vi "UTEXGUI.vi"(8 "ExitSendCmd":bool, 11 "UT340 Controls":T1={"High Pass On"=FALSE, "High Pass Filter (MHz)"=1, "Low Pass On"=FALSE, "Low Pass Filter (MHz)"=20, "PE Gain (dB)"=1, "Voltage"=100, "Pulse Width (ns)"=2.0, "Mode"=FALSE, "PC Gain (dB)"=1, "Trig Source"=FALSE, "Rep Rate (Hz)"=0, "PULSE"=FALSE} {"Low Pass Filter (MHz)" min=20 step=1; "High Pass Filter (MHz)" min=1 max=20 step=1; "Pulse Width (ns)" min=2.0 max=71.75; "Voltage" min=100 max=250 step=2; "PC Gain (dB)" min=0 max=63 step=1; "PE Gain (dB)" min=-6 max=57 step=1}) -> ()   [LabVIEW 2022 SP3]
uses:
  Controls/UTEX Controls.ctl
  PulserGlobals.vi
panel:
  out "error out":errorcluster
  in  "error in":errorcluster
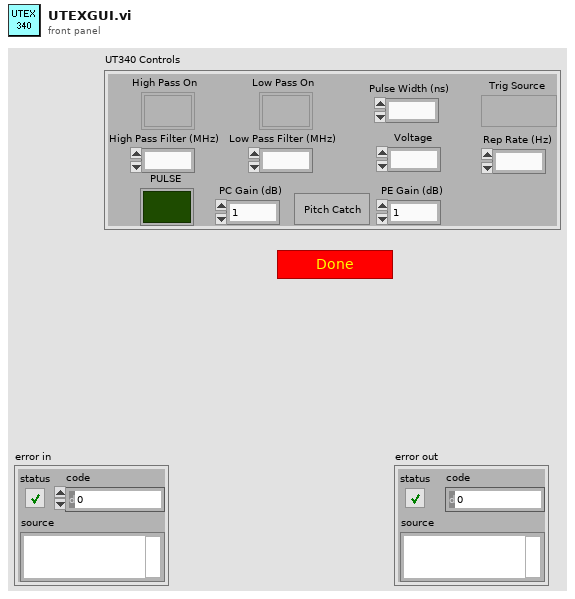
[diagram p1: front panel]
types:
  T1 = typedef "UTEX Controls.ctl" = cluster{"High Pass On":bool, "High Pass Filter (MHz)":i16, "Low Pass On":bool, "Low Pass Filter (MHz)":i16, "PE Gain (dB)":i16, "Voltage":i16, "Pulse Width (ns)":dbl, "Mode":bool, "PC Gain (dB)":i16, "Trig Source":bool, "Rep Rate (Hz)":i16, "PULSE":bool}
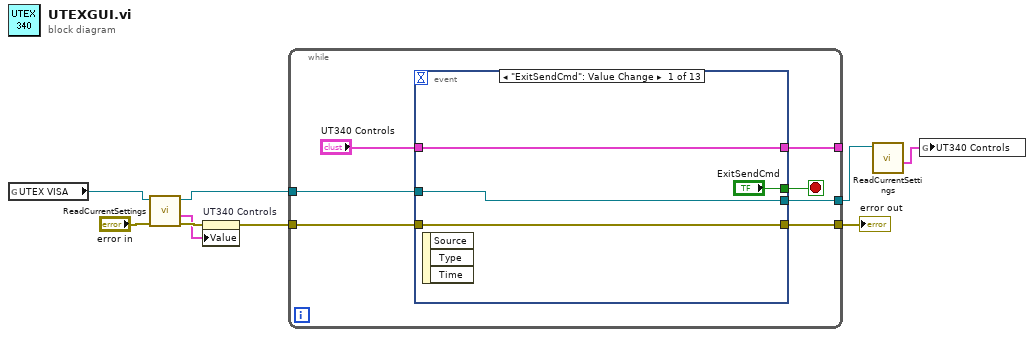
[diagram p0: block diagram]
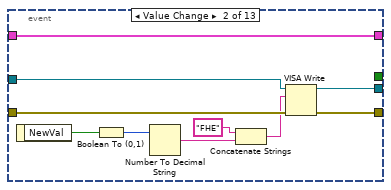
[diagram p2: hidden frame]
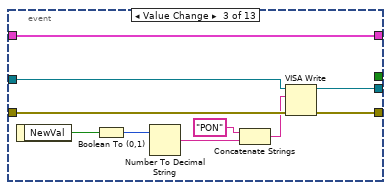
[diagram p3: hidden frame]
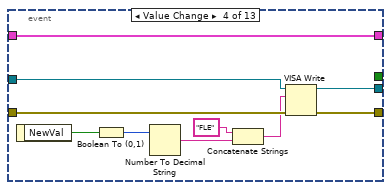
[diagram p4: hidden frame]
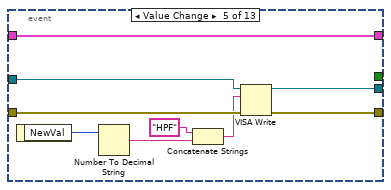
[diagram p5: hidden frame]
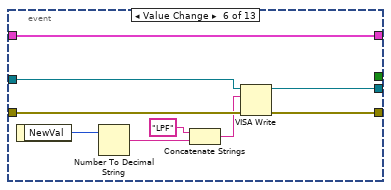
[diagram p6: hidden frame]
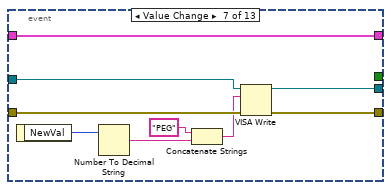
[diagram p7: hidden frame]
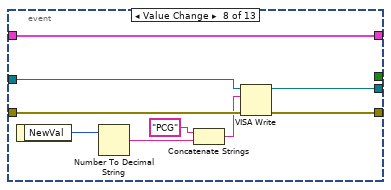
[diagram p8: hidden frame]
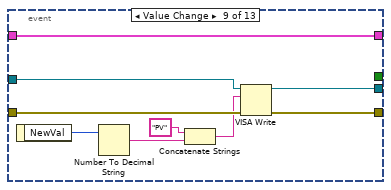
[diagram p9: hidden frame]
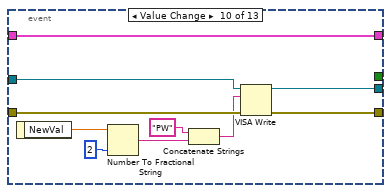
[diagram p10: hidden frame]
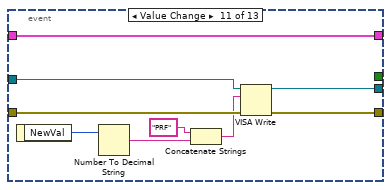
[diagram p11: hidden frame]
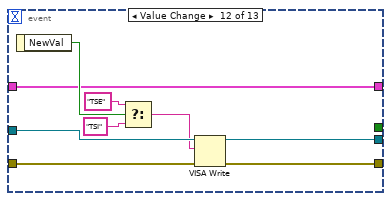
[diagram p12: hidden frame]
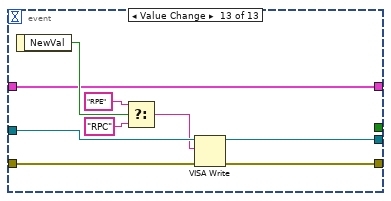
[diagram p13: hidden frame]
diagram:
  n1 = global read "PulserGlobals.vi" "UTEX VISA"() -> (w2:refnum<visa-resource-name>)
  n2 = call "ReadCurrentSettings.vi"("error in (no error)"="error in", "VISA Refnum in"=w2) -> ("error out"=w7:errorcluster, "UT340 Controls"=w4:T1, "VISA Refnum out"=w1:refnum<visa-resource-name>)  [unwired: 7 in]
  n3 = property on="UT340 Controls" class="Clust (strict)"(error in=w7, "Value"=w4) -> (error out=w8:errorcluster)  [unwired: 1 in, 1 out]
  n4 = while {
    tunnel: w8 -> [w15]
    tunnel: w1 -> [w14]
    tunnel: [w13] -> w5
    tunnel: [w12] -> w9
    tunnel: [w10] -> _
    stop <- w11 stop-if-true
    n5 = event shown="[0] \"ExitSendCmd\": Value Change" {
      selector: _ -> [_ _ _ _ _ _ _ _ _ _ _ _ _]
      dyn-events: _ -> [_ _ _ _ _ _ _ _ _ _ _ _ _]
      timeout: _ -> [_ _ _ _ _ _ _ _ _ _ _ _ _]
      tunnel: "UT340 Controls" -> [w17 w21 w31 w41 w51 w60 w69 w78 w87 w96 w106 w115 w124]
      tunnel: w15 -> [w19 w30 w40 w50 w59 w68 w77 w86 w95 w105 w114 w123 w132]
      tunnel: w14 -> [w20 w29 w39 w49 w58 w67 w76 w85 w94 w104 w113 w122 w131]
      tunnel: [w20 w28 w38 w48 w57 w66 w75 w84 w93 w103 w112 w121 w130] -> w13
      tunnel: [w19 w27 w37 w47 w56 w65 w74 w83 w92 w102 w111 w120 w129] -> w12
      tunnel: ["ExitSendCmd" _ _ _ _ _ _ _ _ _ _ _ _] -> w11
      tunnel: [w17 w21 w31 w41 w51 w60 w69 w78 w87 w96 w106 w115 w124] -> w10
      event "ExitSendCmd": Value Change {
        n6 = event-data() -> ()  [unwired: 1 in, 3 out]
      }
      event Value Change {
        n7 = event-data() -> ("NewVal"=w26:bool)  [unwired: 1 in]
        n8 = Boolean To (0,1)(Boolean=w26) -> (0, 1=w22:i16)
        n9 = Number To Decimal String(number=w22) -> (decimal integer string=w24:string)  [unwired: 1 in]
        n10 = Concatenate Strings("FHE" ("string"), w24) -> (w23:string)
        n11 = VISA Write(VISA resource name=w29, write buffer=w23, error in (no error)=w30) -> (VISA resource name out=w28:refnum<visa-resource-name>, error out=w27:errorcluster)  [unwired: 1 out]
      }
      event Value Change {
        n12 = event-data() -> ("NewVal"=w36:bool)  [unwired: 1 in]
        n13 = Boolean To (0,1)(Boolean=w36) -> (0, 1=w32:i16)
        n14 = Number To Decimal String(number=w32) -> (decimal integer string=w34:string)  [unwired: 1 in]
        n15 = Concatenate Strings("PON" ("string"), w34) -> (w33:string)
        n16 = VISA Write(VISA resource name=w39, write buffer=w33, error in (no error)=w40) -> (VISA resource name out=w38:refnum<visa-resource-name>, error out=w37:errorcluster)  [unwired: 1 out]
      }
      event Value Change {
        n17 = event-data() -> ("NewVal"=w46:bool)  [unwired: 1 in]
        n18 = Boolean To (0,1)(Boolean=w46) -> (0, 1=w42:i16)
        n19 = Number To Decimal String(number=w42) -> (decimal integer string=w44:string)  [unwired: 1 in]
        n20 = Concatenate Strings("FLE" ("string"), w44) -> (w43:string)
        n21 = VISA Write(VISA resource name=w49, write buffer=w43, error in (no error)=w50) -> (VISA resource name out=w48:refnum<visa-resource-name>, error out=w47:errorcluster)  [unwired: 1 out]
      }
      event Value Change {
        n22 = event-data() -> ("NewVal"=w55:i16)  [unwired: 1 in]
        n23 = Number To Decimal String(number=w55) -> (decimal integer string=w53:string)  [unwired: 1 in]
        n24 = Concatenate Strings("HPF" ("string"), w53) -> (w52:string)
        n25 = VISA Write(VISA resource name=w58, write buffer=w52, error in (no error)=w59) -> (VISA resource name out=w57:refnum<visa-resource-name>, error out=w56:errorcluster)  [unwired: 1 out]
      }
      event Value Change {
        n26 = event-data() -> ("NewVal"=w64:i16)  [unwired: 1 in]
        n27 = Number To Decimal String(number=w64) -> (decimal integer string=w62:string)  [unwired: 1 in]
        n28 = Concatenate Strings("LPF" ("string"), w62) -> (w61:string)
        n29 = VISA Write(VISA resource name=w67, write buffer=w61, error in (no error)=w68) -> (VISA resource name out=w66:refnum<visa-resource-name>, error out=w65:errorcluster)  [unwired: 1 out]
      }
      event Value Change {
        n30 = event-data() -> ("NewVal"=w73:i16)  [unwired: 1 in]
        n31 = Number To Decimal String(number=w73) -> (decimal integer string=w71:string)  [unwired: 1 in]
        n32 = Concatenate Strings("PEG" ("string"), w71) -> (w70:string)
        n33 = VISA Write(VISA resource name=w76, write buffer=w70, error in (no error)=w77) -> (VISA resource name out=w75:refnum<visa-resource-name>, error out=w74:errorcluster)  [unwired: 1 out]
      }
      event Value Change {
        n34 = event-data() -> ("NewVal"=w82:i16)  [unwired: 1 in]
        n35 = Number To Decimal String(number=w82) -> (decimal integer string=w80:string)  [unwired: 1 in]
        n36 = Concatenate Strings("PCG" ("string"), w80) -> (w79:string)
        n37 = VISA Write(VISA resource name=w85, write buffer=w79, error in (no error)=w86) -> (VISA resource name out=w84:refnum<visa-resource-name>, error out=w83:errorcluster)  [unwired: 1 out]
      }
      event Value Change {
        n38 = event-data() -> ("NewVal"=w91:i16)  [unwired: 1 in]
        n39 = Number To Decimal String(number=w91) -> (decimal integer string=w89:string)  [unwired: 1 in]
        n40 = Concatenate Strings("PV" ("string"), w89) -> (w88:string)
        n41 = VISA Write(VISA resource name=w94, write buffer=w88, error in (no error)=w95) -> (VISA resource name out=w93:refnum<visa-resource-name>, error out=w92:errorcluster)  [unwired: 1 out]
      }
      event Value Change {
        n42 = event-data() -> ("NewVal"=w101:dbl)  [unwired: 1 in]
        n43 = Number To Fractional String(number=w101, precision (6)=i16 2) -> (F-format string=w99:string)  [unwired: 2 in]
        n44 = Concatenate Strings("PW" ("string"), w99) -> (w98:string)
        n45 = VISA Write(VISA resource name=w104, write buffer=w98, error in (no error)=w105) -> (VISA resource name out=w103:refnum<visa-resource-name>, error out=w102:errorcluster)  [unwired: 1 out]
      }
      event Value Change {
        n46 = event-data() -> ("NewVal"=w110:i16)  [unwired: 1 in]
        n47 = Number To Decimal String(number=w110) -> (decimal integer string=w108:string)  [unwired: 1 in]
        n48 = Concatenate Strings("PRF" ("string"), w108) -> (w107:string)
        n49 = VISA Write(VISA resource name=w113, write buffer=w107, error in (no error)=w114) -> (VISA resource name out=w112:refnum<visa-resource-name>, error out=w111:errorcluster)  [unwired: 1 out]
      }
      event Value Change {
        n50 = event-data() -> ("NewVal"=w119:bool)  [unwired: 1 in]
        n51 = Select(t="TSE" ("string"), s=w119, f="TSI") -> (s? t:f=w118:string)
        n52 = VISA Write(VISA resource name=w122, write buffer=w118, error in (no error)=w123) -> (VISA resource name out=w121:refnum<visa-resource-name>, error out=w120:errorcluster)  [unwired: 1 out]
      }
      event Value Change {
        n53 = event-data() -> ("NewVal"=w128:bool)  [unwired: 1 in]
        n54 = Select(t="RPE" ("string"), s=w128, f="RPC") -> (s? t:f=w127:string)
        n55 = VISA Write(VISA resource name=w131, write buffer=w127, error in (no error)=w132) -> (VISA resource name out=w130:refnum<visa-resource-name>, error out=w129:errorcluster)  [unwired: 1 out]
      }
    }
  }
  "error out" <- w9
  n56 = call "ReadCurrentSettings.vi"("VISA Refnum in"=w5) -> ("UT340 Controls"=w3:T1)  [unwired: 8 in, 2 out]
  n57 = global write "PulserGlobals.vi" "UT340 Controls"(w3) -> ()
